vi "Distance to RPM and Angle.vi"(10 "distance (m)":dbl) -> (2 "Angle for Hood":dbl, 3 "speed of flywheel  (m/s)":dbl)   [LabVIEW 2016]
panel:
  out "Vx":dbl
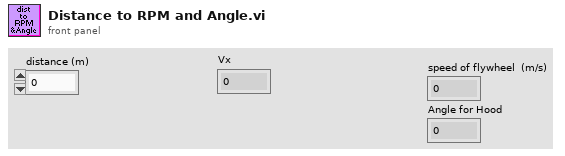
[diagram p1: front panel]
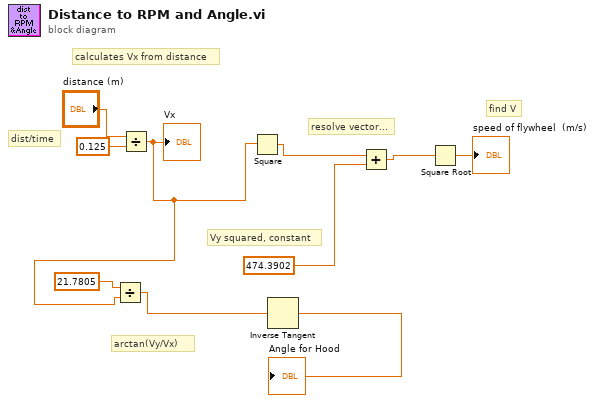
[diagram p0: block diagram]
diagram:
  # "arctan(Vy/Vx)"
  # "resolve vector..."
  # "dist/time"
  # "find V"
  # "Vy squared, constant"
  # "calculates Vx from distance"
  n1 = Divide(x="distance (m)", y=0.125) -> (x/y=w3:dbl)
  "Vx" <- w3
  n2 = Divide(x=21.7805, y=w3) -> (x/y=w2:dbl)
  n3 = Square(x=w3) -> (x^2=w8:dbl)
  n4 = Inverse Tangent(1:w2) -> (0:→"Angle for Hood":dbl)
  n5 = Add(x=w8, y=474.3902 ("Vy")) -> (x+y=w6:dbl)
  n6 = Square Root(x=w6) -> (sqrt(x)=→"speed of flywheel  (m/s)":dbl)
